vi "FPGA.vi"() -> ()   [LabVIEW 2018]
uses:
  <vilib>/rvi/Emulation/niFpgaGetClockAttributes.vi
  <vilib>/rvi/Emulation/niFpgaSctlEmulationGetInTimedLoop.vi
  <vilib>/rvi/Emulation/niFpgaEmulationReportErrorSimple.vi
  <vilib>/rvi/Emulation/niFpgaProcessEmulError.vi
  <vilib>/rvi/Emulation/niFpgaCriticalErrorInLSC.vi
  <vilib>/rvi/eio/common/nirviEmuTemplateMethod_errors.vi
  <vilib>/eio/EIONode/EIONode.xnode
panel:
  in  "tape_sensor_threshold":fxp<+/-,21,-4>=0.004999995231628418 format="%#_27g"
  in  "distance_per_tape":sgl=100.0
  out "samples_taken":i32
  in  "reset_distance":i16
  out "distance":sgl
  out "tape_sensor_raw":fxp<+/-,21,-4>
  out "pwm0_signal":bool
  in  "pwm0_duty_cycle":sgl
  in  "pwm0_frequency":sgl
  in  "pwm0_enable":bool
  # "PWM0"
  # "Tape Sensor"
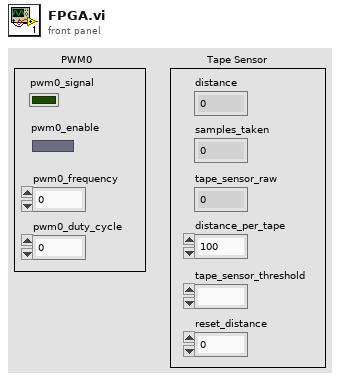
[diagram p1: front panel]
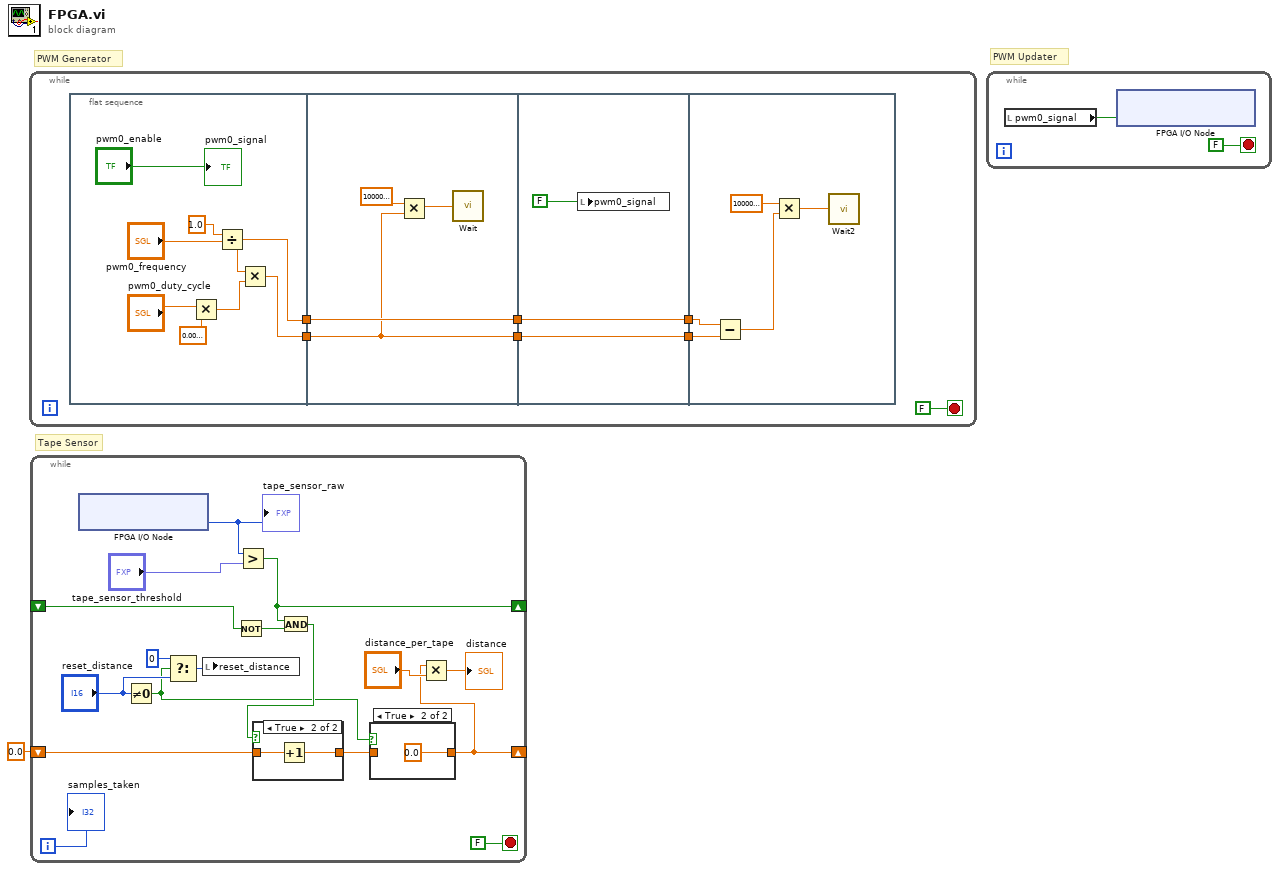
[diagram p0: block diagram]
diagram:
  # "Tape Sensor"
  # "PWM Updater"
  # "PWM Generator"
  n1 = while {
    stop <- FALSE stop-if-true
    n2 = flat-sequence {
      tunnel: [w11] -> w8
      tunnel: [w10] -> w7
      tunnel: w8 -> [w19]
      tunnel: w7 -> [w20]
      tunnel: [w19] -> w6
      tunnel: [w20] -> w5
      tunnel: w6 -> [w23]
      tunnel: w5 -> [w22]
      tunnel: [w23] -> w4
      tunnel: [w22] -> w3
      tunnel: w4 -> [w28]
      tunnel: w3 -> [w27]
      frame #0 {
        n3 = Multiply(x=sgl 0.01, y="pwm0_duty_cycle") -> (x*y=w14:sgl)
        n4 = Divide(x=sgl 1.0, y="pwm0_frequency") -> (x/y=w10:sgl)
        n5 = Multiply(x=w10, y=w14) -> (x*y=w11:sgl)
        "pwm0_signal" <- "pwm0_enable"
      }
      frame #1 {
        n6 = Multiply(x=sgl 1000000.0, y=w19) -> (x*y=w17:sgl)
        n7 = call "Wait"("Count(uSec)"=w17) -> ()  [unwired: 1 out]
      }
      frame #2 {
        n8 = local write "pwm0_signal"(FALSE ("ConnectorC/DIO7")) -> ()
      }
      frame #3 {
        n9 = Subtract(x=w27, y=w28) -> (x-y=w26:sgl)
        n10 = Multiply(x=sgl 1000000.0, y=w26) -> (x*y=w24:sgl)
        n11 = call "Wait2"("Count(uSec)"=w24) -> ()  [unwired: 1 out]
      }
    }
  }
  n12 = while {
    shift-right: [w29] -> _
    shift-left: sgl 0.0 -> [w32]
    shift-right: [w43] -> _
    shift-left: _ -> [w45]
    i -> [w42]
    stop <- FALSE stop-if-true
    n13 = xnode "FPGA I/O Node"() -> ("ConnectorC/AI0"=w41:i16)  [unwired: 1 in, 1 out]
    "tape_sensor_raw" <- w41
    n14 = Not Equal To 0?(x="reset_distance") -> (x != 0?=w31:bool)
    n15 = Select(t=i16 0, s=w31, f="reset_distance") -> (s? t:f=w36:i16)
    n16 = local write "reset_distance"(w36) -> ()
    n17 = Not(x=w45) -> (.not. x?=w44:bool)
    n18 = Greater?(x=w41, y="tape_sensor_threshold") -> (0:w43:bool)
    n19 = And(x=w43, y=w44) -> (x .and. y?=w33:bool)
    n20 = case shown="True" w33 {
      tunnel: w32 -> [w48 w50]
      tunnel: [w48 w49] -> w30
      frame False {
      }
      frame True {
        n21 = Increment(x=w50) -> (x+1=w49:sgl)
      }
    }
    n22 = case shown="True" w31 {
      tunnel: w30 -> [w46 _]
      tunnel: [w46 sgl 0.0] -> w29
      frame False {
      }
      frame True {
      }
    }
    n23 = Multiply(x=w29, y="distance_per_tape") -> (x*y=→"distance":sgl)
    "samples_taken" <- w42
  }
  n24 = while {
    stop <- FALSE stop-if-true
    n25 = local read "pwm0_signal"() -> (w52:bool)
    n26 = xnode "FPGA I/O Node"("ConnectorC/DIO7"=w52) -> ()  [unwired: 1 in, 1 out]
  }
